vi "Open expanded image window.vi"(7 "Button":u16, 11 "Image name":string) -> ()   [LabVIEW 2013]
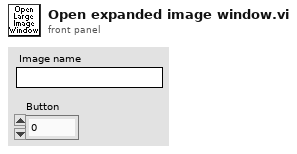
[diagram p1: front panel]
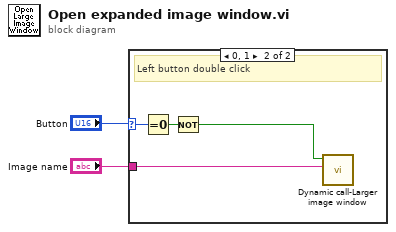
[diagram p0: block diagram]
diagram:
  n1 = case shown="0, 1" "Button" {
    selector: "Button" -> [_ w5]
    tunnel: "Image name" -> [_ w6]
    frame Default {
    }
    frame 0, 1 {
      # "Left button double click"
      n2 = Equal To 0?(x=w5) -> (x = 0?=w4:bool)
      n3 = Not(x=w4) -> (.not. x?=w3:bool)
      n4 = call "Dynamic call-Larger image window.vi"("Image name"=w6, "Open maximised"=w3) -> ()  [unwired: 9 in, 1 out]
    }
  }
